vi "GHV232 CRAB Version Response.vi"(11 "Recieve Packet":string) -> (1 "Message":string)   [LabVIEW 2017]
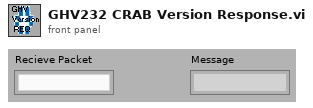
[diagram p1: front panel]
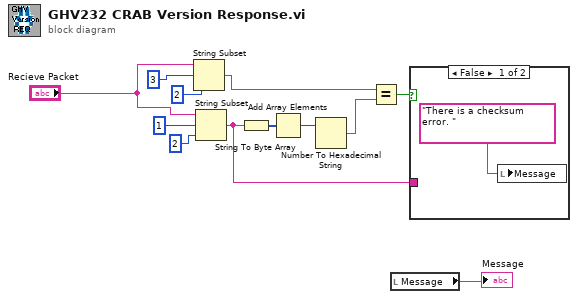
[diagram p0: block diagram]
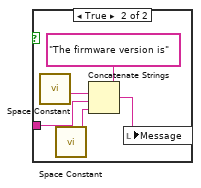
[diagram p2: hidden frame]
diagram:
  n1 = String Subset(string="Recieve Packet", offset (0)=3, length (rest)=2) -> (substring=w8:string)
  n2 = String Subset(string="Recieve Packet", offset (0)=1, length (rest)=2) -> (substring=w3:string)
  n3 = String To Byte Array(string=w3) -> (unsigned byte array=w9:u8[])
  n4 = Add Array Elements(numeric array=w9) -> (sum=w7:u8)
  n5 = Number To Hexadecimal String(2:w7) -> (0:w6:string)  [unwired: 1 in]
  n6 = Equal?(x=w8, y=w6) -> (x = y?=w5:bool)
  n7 = local read "Message"() -> (→"Message":string)
  n8 = case shown="False" w5 {
    tunnel: w3 -> [_ w16]
    frame False {
      n9 = local write "Message"("There is a checksum error. ") -> ()
    }
    frame True {
      n10 = call <vilib>:"Space Constant.vi"() -> ("String"=w17:string)
      n11 = call <vilib>:"Space Constant.vi"() -> ("String"=w14:string)
      n12 = Concatenate Strings("The firmware version is", w17, w16, w14) -> (w15:string)
      n13 = local write "Message"(w15) -> ()
    }
  }
